vi "Updater Convert TDMS File 5.0 to 5.1.vi"(5 "Current Version":string, 6 "Connection Refnum In":T1, 7 "Previous Version":string, 8 "error in (no error)":errorcluster, 11 "TDMS Path":path) -> (0 "error out":errorcluster, 3 "Conversion Time (ms)":u32, 4 "Connection Refnum Out":T1)   [LabVIEW 2011]
uses:
  SI.LIB/ODBC/SQL Controls/Connection Refnum.ctl
panel:
  out "Group Names":string[](array[string])
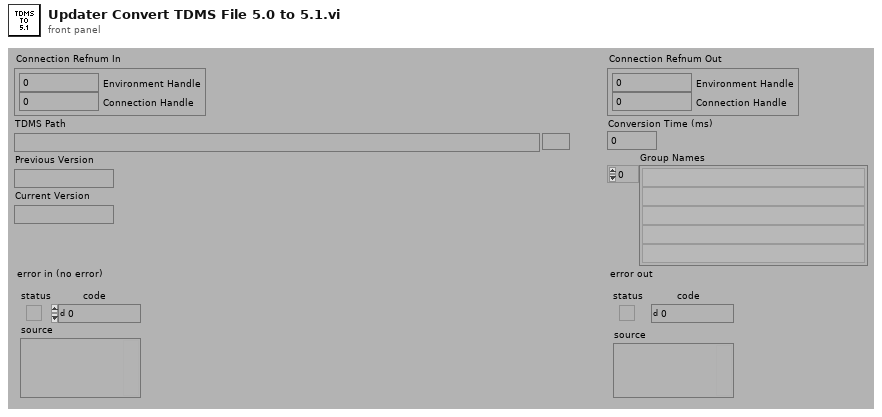
[diagram p1: front panel]
types:
  T1 = typedef "Connection Refnum.ctl" = cluster{"Environment Handle":i32, "Connection Handle":i32}
  T2 = enum16{"open", "open or create", "create or replace", "create", "open (read-only)"}
  T3 = typedef "Field Record.ctl" = cluster{"ixField":i32, "iSequenceOrder":i32, "sxFieldId":string, "sxSequenceId":string, "sDisplayName":string, "sValue":string, "sUnits":string, "nDataType":T4, "nNextItem":T5, "fSystem":bool, "fSystemValue":bool, "fRequired":bool, "fSetAtTest":bool, "fTestField":bool, "fDeleted":bool, "fIndexed":bool, "fFreeList":bool}
  T4 = typedef "Field DataTypes.ctl" = enum32{"text", "numeric", "list", "timestamp", "boolean"}
  T5 = typedef "Field NextItem.ctl" = enum32{"Reset", "Retain", "Auto-Increment"}
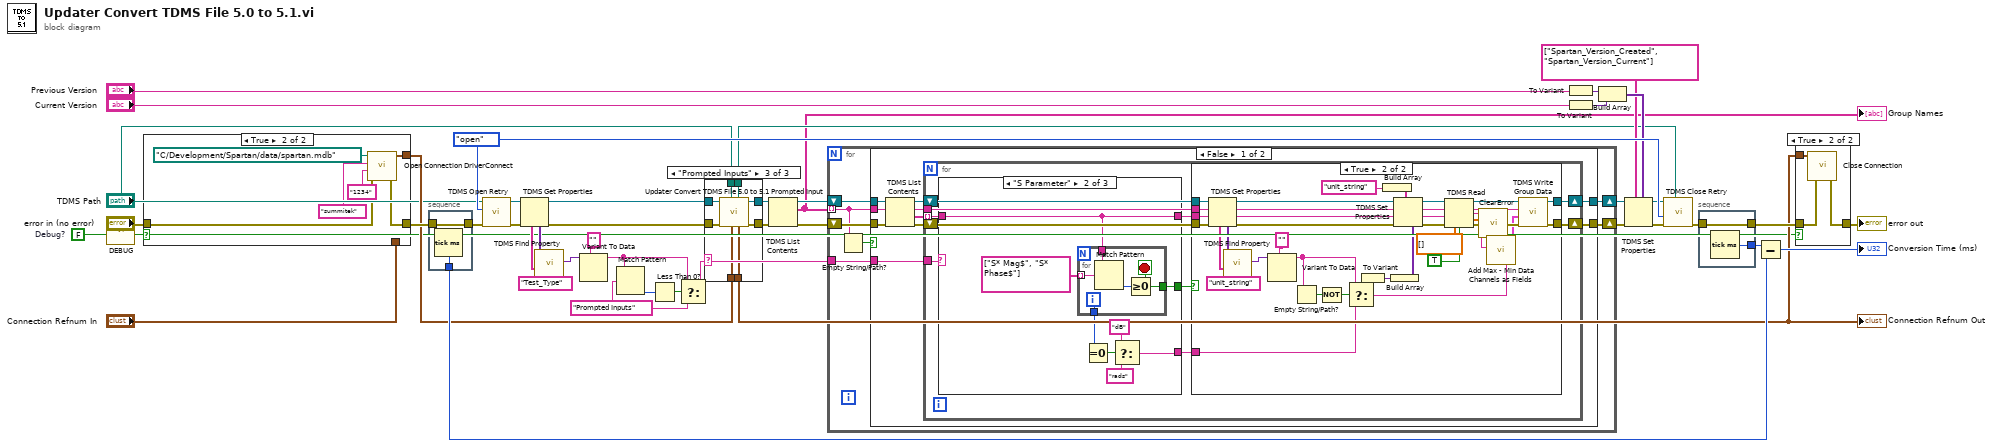
[diagram p0: block diagram]
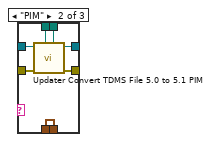
[diagram p5: hidden frame]
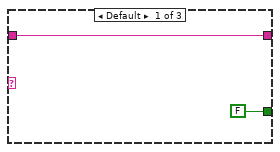
[diagram p7: hidden frame]
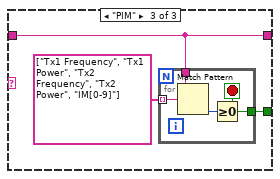
[diagram p8: hidden frame]
diagram:
  w13 = FALSE  # Debug?
  w16 = "Prompted Inputs" ("element")
  w33 = T2."open" ("operation (0:open)")
  n1 = call "DEBUG.vi"("Dev DEBUG? (f)"=w13) -> ("DEBUG?"=w5:bool)  [unwired: 1 in, 5 out]
  n2 = case shown="True" w5 {
    tunnel: "error in (no error)" -> [w47 w52]
    tunnel: [w47 w51] -> w11
    tunnel: [w48 w50] -> w9
    tunnel: "Connection Refnum In" -> [w48 _]
    frame False {
    }
    frame True {
      n3 = call "Open Connection DriverConnect.vi"("error in (no error)"=w52, "Password (\"\")"="1234" ("Username (\"\")"), "Username (\"\")"="summitek" ("Username (\"\")"), "ODBC Database (\"\")"=path "C:/Development/Spartan/data/spartan.mdb" ("ODBC Database (\"\")")) -> ("error out"=w51:errorcluster, "Connection Refnum"=w50:T1)  [unwired: 3 out]
    }
  }
  n4 = stacked-sequence {
    tunnel: w11 -> [w56]
    tunnel: [w56] -> w45
    tunnel: [w55] -> w43
    frame #0 {
      n5 = Tick Count (ms)() -> (millisecond timer value=w55:u32)
    }
  }
  n6 = call "TDMS Open Retry.vi"("error in (no error)"=w45, "Operation (0:open)"=w33, "Path"="TDMS Path") -> ("error out"=w40:errorcluster, "TDMS File Ref"=w39:refnum<k34>)  [unwired: 1 in, 6 out]
  n7 = TDMS Get Properties(8:w40, 11:w39) -> (0:w31:errorcluster, 3:w32:refnum<k34>, 4:w37:variant[], 6:w36:string[])  [unwired: 6 out]
  n8 = call "TDMS Find Property.vi"("Property Name"="Test_Type" ("element"), "Property Names"=w36, "Property Values"=w37) -> ("Property Value"=w35:variant)  [unwired: 5 out]
  n9 = Variant To Data(type="" ("element"), Variant=w35) -> (data=w15:string)  [unwired: 1 in, 1 out]
  n10 = Match Pattern(string=w15, regular expression=w16) -> (offset past match=w18:i32)  [unwired: 4 out]
  n11 = Less Than 0?(x=w18) -> (x < 0?=w17:bool)
  n12 = Select(t=w15, s=w17, f=w16) -> (s? t:f=w14:string)
  n13 = case shown="\"Prompted Inputs\"" w14 {
    tunnel: w32 -> [w60 w65 w73]
    tunnel: w31 -> [w59 w67 w75]
    tunnel: [w60 w64 w72] -> w30
    tunnel: [w59 w66 w74] -> w29
    tunnel: "TDMS Path" -> [w57 w63 w71]
    tunnel: w9 -> [w58 w62 w70]
    tunnel: [w58 w62 w69] -> w6
    tunnel: [w57 w61 w68] -> w3
    frame Default {
    }
    frame "PIM" {
      n14 = call "Updater Convert TDMS File 5.0 to 5.1 PIM.vi"("TDMS Path In"=w63, "error in (no error)"=w67, "TDMS File Ref"=w65) -> ("error out"=w66:errorcluster, "TDMS File Ref"=w64:refnum<k34>, "TDMS Path Out"=w61:path)  [unwired: 6 out]
    }
    frame "Prompted Inputs" {
      n15 = call "Updater Convert TDMS File 5.0 to 5.1 Prompted Input.vi"("Connection Refnum In"=w70, "TDMS Path In"=w71, "error in (no error)"=w75, "TDMS File Ref"=w73) -> ("error out"=w74:errorcluster, "TDMS File Ref"=w72:refnum<k34>, "Connection Refnum Out"=w69:T1, "TDMS Path Out"=w68:path)  [unwired: 4 out]
    }
  }
  "Connection Refnum Out" <- w6
  n16 = TDMS List Contents(4:w29, 7:w30) -> (0:w46:errorcluster, 2:w2:string[], 3:w41:refnum<k34>)  [unwired: 2 out]
  "Group Names" <- w2
  n17 = for {
    shift-right: [w76] -> w25
    shift-left: w46 -> [w81]
    tunnel: w2 -> [w80] mode=indexing
    shift-right: [w77] -> w28
    shift-left: w41 -> [w82]
    tunnel: w14 -> [w78]
    n18 = Empty String/Path?(string/path=w80) -> (empty?=w79:bool)
    n19 = case shown="False" w79 {
      tunnel: w82 -> [w92 w165]
      tunnel: w81 -> [w91 w164]
      tunnel: [w85 w164] -> w76
      tunnel: w80 -> [w90 _]
      tunnel: [w86 w165] -> w77
      tunnel: w78 -> [w89 _]
      frame False {
        n20 = TDMS List Contents(4:w91, 6:w90, 7:w92) -> (0:w88:errorcluster, 1:w83:string[], 2:w84:string, 3:w87:refnum<k34>)
        n21 = for {
          tunnel: w89 -> [w102]
          tunnel: w83 -> [w94] mode=indexing
          tunnel: w84 -> [w96]
          shift-right: [w98] -> w86
          shift-left: w87 -> [w100]
          shift-right: [w97] -> w85
          shift-left: w88 -> [w101]
          n22 = case shown="\"S Parameter\"" w102 {
            tunnel: [FALSE w150 w159] -> w99
            tunnel: [_ w145 _] -> w95
            tunnel: w94 -> [w142 w144 w158]
            tunnel: [w142 w144 w158] -> w93
            frame Default {
            }
            frame "S Parameter" {
              n23 = for {
                tunnel: string[] ["S* Mag$", "S* Phase$"] -> [w156] mode=indexing
                tunnel: w144 -> [w155]
                tunnel: [w153] -> w150
                tunnel: [w152] -> w146
                i -> [w152]
                stop <- w153 stop-if-true
                n24 = Match Pattern(string=w155, regular expression=w156) -> (offset past match=w154:i32)  [unwired: 4 out]
                n25 = Greater Or Equal To 0?(x=w154) -> (x >= 0?=w153:bool)
              }
              n26 = Equal To 0?(x=w146) -> (x = 0?=w147:bool)
              n27 = Select(t="dB" ("regular expression"), s=w147, f="rads") -> (s? t:f=w145:string)
            }
            frame "PIM" {
              n28 = for {
                tunnel: string[] ["Tx1 Frequency", "Tx1 Power", "Tx2 Frequency", "Tx2 Power", "IM[0-9]"] -> [w163] mode=indexing
                tunnel: w158 -> [w162]
                tunnel: [w160] -> w159
                stop <- w160 stop-if-true
                n29 = Match Pattern(string=w162, regular expression=w163) -> (offset past match=w161:i32)  [unwired: 4 out]
                n30 = Greater Or Equal To 0?(x=w161) -> (x >= 0?=w160:bool)
              }
            }
          }
          n31 = case shown="True" w99 {
            tunnel: w101 -> [w103 w124]
            tunnel: w100 -> [w104 w127]
            tunnel: [w104 w133] -> w98
            tunnel: [w103 w134] -> w97
            tunnel: w96 -> [_ w126]
            tunnel: w93 -> [_ w125]
            tunnel: w95 -> [_ w120]
            frame False {
            }
            frame True {
              n32 = TDMS Get Properties(8:w124, 9:w125, 10:w126, 11:w127) -> (0:w116:errorcluster, 1:w117:string, 2:w118:string, 3:w119:refnum<k34>, 4:w129:variant[], 6:w130:string[])  [unwired: 2 out]
              n33 = call "TDMS Find Property.vi"("Property Name"="unit_string" ("element"), "Property Names"=w130, "Property Values"=w129) -> ("Property Value"=w131:variant)  [unwired: 5 out]
              n34 = Variant To Data(type="" ("element"), Variant=w131) -> (data=w121:string)  [unwired: 1 in, 1 out]
              n35 = Empty String/Path?(string/path=w121) -> (empty?=w123:bool)
              n36 = Not(x=w123) -> (.not. x?=w122:bool)
              n37 = Select(t=w121, s=w122, f=w120) -> (s? t:f=w111:string)
              n38 = To Variant(anything=w111) -> (Variant=w110:variant)
              n39 = Build Array("unit_string" ("element")) -> (w107:string[])
              n40 = Build Array(w110) -> (w109:variant[])
              n41 = TDMS Set Properties(5:w109, 7:w107, 8:w116, 9:w117, 10:w118, 11:w119) -> (0:w114:errorcluster, 1:w112:string, 2:w113:string, 3:w115:refnum<k34>)
              n42 = TDMS Read(0:w115, 5:w113, 7:w112, 11:w114, 12:dbl[] [] ("Data Channel"), 13:TRUE ("return channels in file order? (F)")) -> (4:w138:refnum<k34>, 6:w135:string, 8:w139:string, 10:w140:dbl[], 15:w106:errorcluster)  [unwired: 2 in, 1 out]
              n43 = call <vilib>:"ClearError.vi"("error in (no error)"=w106) -> ("error out"=w137:errorcluster)
              n44 = call "Add Max - Min Data Channels as Fields.vi"("Units"=w111, "Data Channel"=w140, "Channel Name"=w139) -> ("Fields Out"=w136:T3[])  [unwired: 1 in, 7 out]
              n45 = call "TDMS Write Group Data.vi"("error in (no error)"=w137, "Fields Array"=w136, "Channel Group"=w135, "TDMS File Ref"=w138) -> ("error out"=w134:errorcluster, "TDMS File Ref"=w133:refnum<k34>)  [unwired: 6 out]
            }
          }
        }
      }
      frame True {
      }
    }
  }
  n46 = To Variant(anything="Previous Version") -> (Variant=w21:variant)
  n47 = To Variant(anything="Current Version") -> (Variant=w22:variant)
  n48 = Build Array(w21, w22) -> (w20:variant[])
  n49 = TDMS Set Properties(5:w20, 7:string[] ["Spartan_Version_Created", "Spartan_Version_Current"], 8:w25, 11:w28) -> (0:w26:errorcluster, 3:w27:refnum<k34>)  [unwired: 4 out]
  n50 = call "TDMS Close Retry.vi"("TDMS Path"=w3, "error in (no error)"=w26, "Operation (0:open)"=w33, "TDMS File Ref"=w27) -> ("error out"=w1:errorcluster)  [unwired: 1 in, 6 out]
  n51 = stacked-sequence {
    tunnel: w1 -> [w167]
    tunnel: [w167] -> w8
    tunnel: [w166] -> w44
    frame #0 {
      n52 = Tick Count (ms)() -> (millisecond timer value=w166:u32)
    }
  }
  n53 = Subtract(x=w44, y=w43) -> (x-y=→"Conversion Time (ms)":u32)
  n54 = case shown="True" w5 {
    tunnel: w8 -> [w168 w171]
    tunnel: [w168 w170] -> w7
    tunnel: w6 -> [_ w169]
    frame False {
    }
    frame True {
      n55 = call "Close Connection.vi"("error in (no error)"=w171, "Connection Refnum"=w169) -> ("error out"=w170:errorcluster)  [unwired: 5 out]
    }
  }
  "error out" <- w7
